vi "test_timer.vi"() -> ()   [LabVIEW 2018]
panel:
  out "pause time":dbl format="%.1f"
  out "run time":dbl format="%.1f"
  out "total time":dbl format="%.1f"
  in  "reset":bool
  in  "pause":bool
  in  "dt":u32
  in  "정지":bool
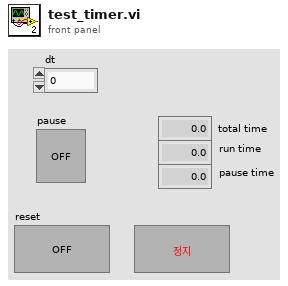
[diagram p1: front panel]
types:
  T1 = cluster{"total time":dbl, "run time":dbl, "pause time":dbl}
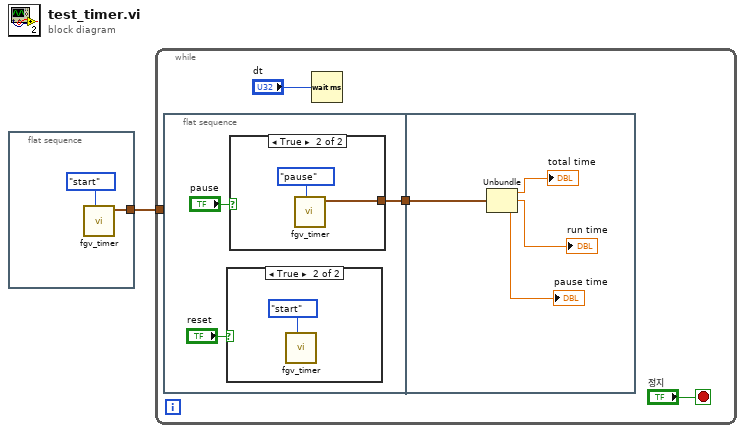
[diagram p0: block diagram]
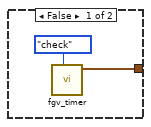
[diagram p3: hidden frame]
diagram:
  n1 = flat-sequence {
    tunnel: [w2] -> w1
    frame #0 {
      n2 = call "fgv_timer.vi"("cmd"=enum16{"check", "start", "pause"}."start") -> ("time_status_out"=w2:T1)  [unwired: 8 in, 2 out]
    }
  }
  n3 = while {
    tunnel: w1 -> [_]
    stop <- "정지" stop-if-true
    n4 = flat-sequence {
      tunnel: [w7] -> w4
      tunnel: w4 -> [w15]
      frame #0 {
        n5 = case shown="True" "reset" {
          frame False {
          }
          frame True {
            n6 = call "fgv_timer.vi"("cmd"=enum16{"check", "start", "pause"}."start") -> ()  [unwired: 8 in, 3 out]
          }
        }
        n7 = case shown="True" "pause" {
          tunnel: [w11 w13] -> w7
          frame False {
            n8 = call "fgv_timer.vi"("cmd"=enum16{"check", "start", "pause"}."check") -> ("time_status_out"=w11:T1)  [unwired: 8 in, 2 out]
          }
          frame True {
            n9 = call "fgv_timer.vi"("cmd"=enum16{"check", "start", "pause"}."pause") -> ("time_status_out"=w13:T1)  [unwired: 8 in, 2 out]
          }
        }
      }
      frame #1 {
        n10 = Unbundle(w15) -> ("total time"=→"total time":dbl, "run time"=→"run time":dbl, "pause time"=→"pause time":dbl)
      }
    }
    n11 = Wait (ms)(milliseconds to wait="dt") -> ()  [unwired: 1 out]
  }
